vi "Unflatten Asynchronous Execution Units.vi"(8 "error in":errorcluster, 11 "Compiled Asynchronous Execution Units":T2[](array[typedef])) -> (0 "error out":errorcluster, 3 "Asynchronous Execution Units":T1[](array[typedef]))   [LabVIEW 2020, in "AIM ARINC 429 Engine.lvlib" / "Custom Device.lvlib"]
uses:
  Custom Device.lvlib
  Asynchronous Execution Unit Compiled Information.ctl
  Asynchronous Execution Unit Runtime Information.ctl
  Interfaces/Execution Unit/Execution Unit.lvclass
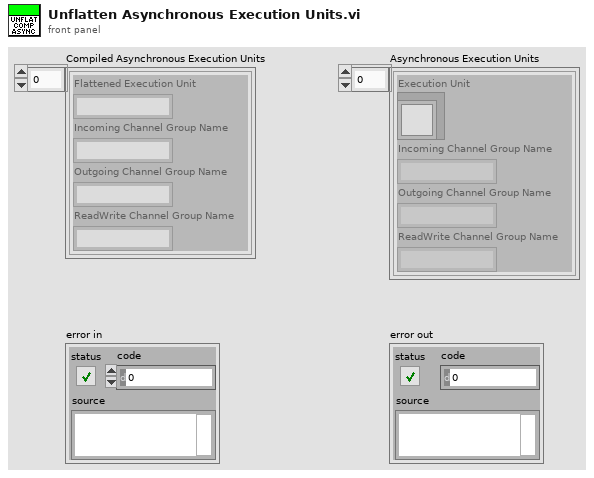
[diagram p1: front panel]
types:
  T1 = typedef "AIM ARINC 429 Engine.lvlib/Custom Device.lvlib/Asynchronous Execution Unit Runtime Information.ctl" = cluster{"Execution Unit":refnum<class "Execution Unit.lvclass">, "Incoming Channel Group Name":string, "Outgoing Channel Group Name":string, "ReadWrite Channel Group Name":string}
  T2 = typedef "AIM ARINC 429 Engine.lvlib/Custom Device.lvlib/Asynchronous Execution Unit Compiled Information.ctl" = cluster{"Flattened Execution Unit":string, "Incoming Channel Group Name":string, "Outgoing Channel Group Name":string, "ReadWrite Channel Group Name":string}
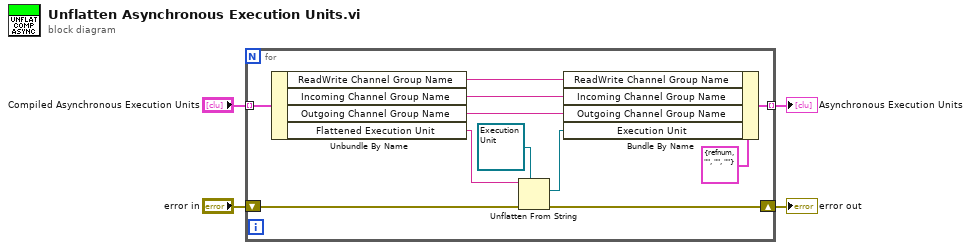
[diagram p0: block diagram]
diagram:
  n1 = for {
    tunnel: "Compiled Asynchronous Execution Units" -> [w12] mode=indexing
    tunnel: [w8] -> w1 mode=indexing
    shift-right: [w14] -> w3
    shift-left: "error in" -> [w15]
    n2 = Unbundle By Name(w12) -> ("ReadWrite Channel Group Name"=w5:string, "Incoming Channel Group Name"=w7:string, "Outgoing Channel Group Name"=w6:string, "Flattened Execution Unit"=w9:string)
    n3 = Unflatten From String(type=refnum<class "Execution Unit.lvclass"> refnum ("Communication Bus Template Interfaces:Execution Unit.lvlib:Execution Unit.lvclass"), binary string=w9, error in (no error)=w15) -> (value=w10:refnum<class "Execution Unit.lvclass">, error out=w14:errorcluster)  [unwired: 2 in, 1 out]
    n4 = Bundle By Name(cluster=T1 {"Execution Unit"=refnum, "Incoming Channel Group Name"="", "Outgoing Channel Group Name"="", "ReadWrite Channel Group Name"=""} ("Asynchronous Execution Unit Runtime Information"), "ReadWrite Channel Group Name"=w5, "Incoming Channel Group Name"=w7, "Outgoing Channel Group Name"=w6, "Execution Unit"=w10) -> (w8:T1)
  }
  "error out" <- w3
  "Asynchronous Execution Units" <- w1
